vi "Control Panel.vi"(8 "error in (no error)":errorcluster, 11 "Fake Lakeshore Gaussmeter in":refnum<class "Lakeshore Gaussmeter.lvclass">) -> (0 "error out":errorcluster, 3 "Fake Lakeshore Gaussmeter out":refnum<class "Lakeshore Gaussmeter.lvclass">)   [LabVIEW 2017, in "Lakeshore Gaussmeter.lvclass"]
doc: "(Dynamic) A user-level application that simulates the physical front panel of the Instrument. Provide the user with buttons to manually control features of the instrument, and provide indicators of its current state."
uses:
  Lakeshore Gaussmeter.lvclass
  Lakeshore Gaussmeter.lvclass/Lakeshore Gaussmeter.ctl
  Utility Classes/Scannable/Scannable.lvclass
panel:
  in  "Auto Range Set (F: Off)":bool
  in  "Range Set (0: 1 - Lowest)":u16(ring) items=["1 - Lowest", "2", "3", "4", "5 - Highest"]
  out "Auto Range (F: Off)":bool
  out "Range (0: 1 - Lowest)":u16(ring) items=["1 - Lowest", "2", "3", "4", "5 - Highest"]
  in  "Set Units":bool
  in  "Field Control Mode Set":u16(ring) items=["Off", "Closed Loop PI", "Manual"]
  out "Field Control Mode":u16(ring) items=["Off", "Closed Loop PI", "Manual"]
  in  "Control Slope Limit Set (10.00000E+0)":dbl=10.0
  in  "Ramp Rate Set (3.50000E+3)":dbl=3500.0
  in  "Integral (reset) Set (1.00000E+0)":dbl=1.0
  in  "Proportional (gain) Set (10.00000E+0)":dbl=10.0
  in  "Setpoint Set":dbl min=0.0 max=13600.0
  out "Control Slope Limit":dbl
  out "Ramp Rate":dbl
  out "Integral (reset)":dbl
  out "Proportional (gain)":dbl
  out "Setpoint Ramping?":bool
  out "Setpoint":dbl
  in  "Field Units Set (0: Gauss)":u16(ring) items=["Gauss", "Tesla", "Oersted", "Amp/meter"]
  out "Field Units":u16(ring) items=["Gauss", "Tesla", "Oersted", "Amp/meter"]
  out "Field Reading":dbl
  in  "Reset":bool
  in  "Set Values":bool
  in  "Read to Control":bool
  in  "Read":bool
  in  "stop":bool
  in  "Copy actual to set":bool
  in  "Populate fields with member data":bool
  # "Not higher than 1.36T =13600G!"
  # "Inconsistent bug: set this to 10 in gauss mode (not 0.01) if field doesn't change when set."
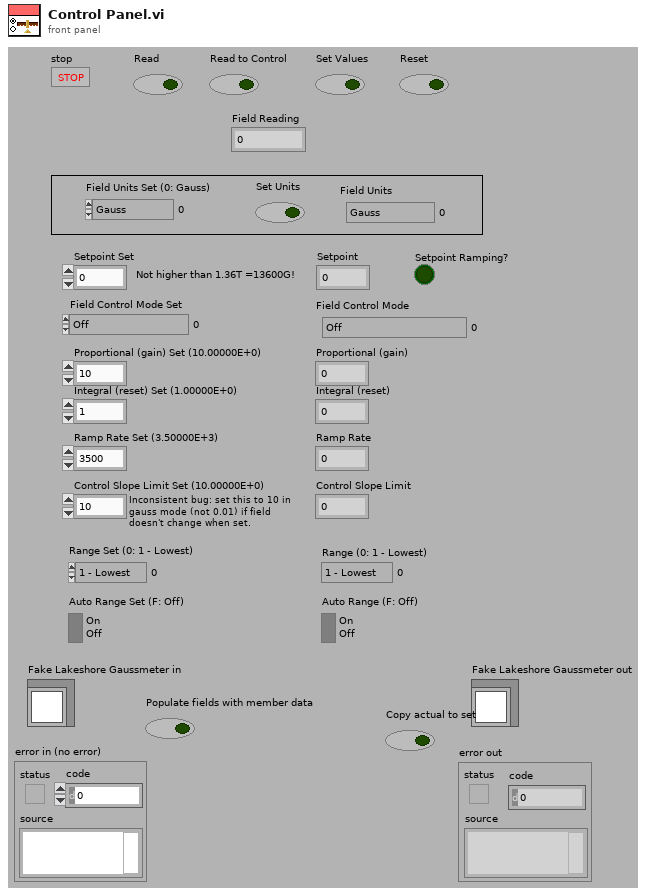
[diagram p1: front panel]
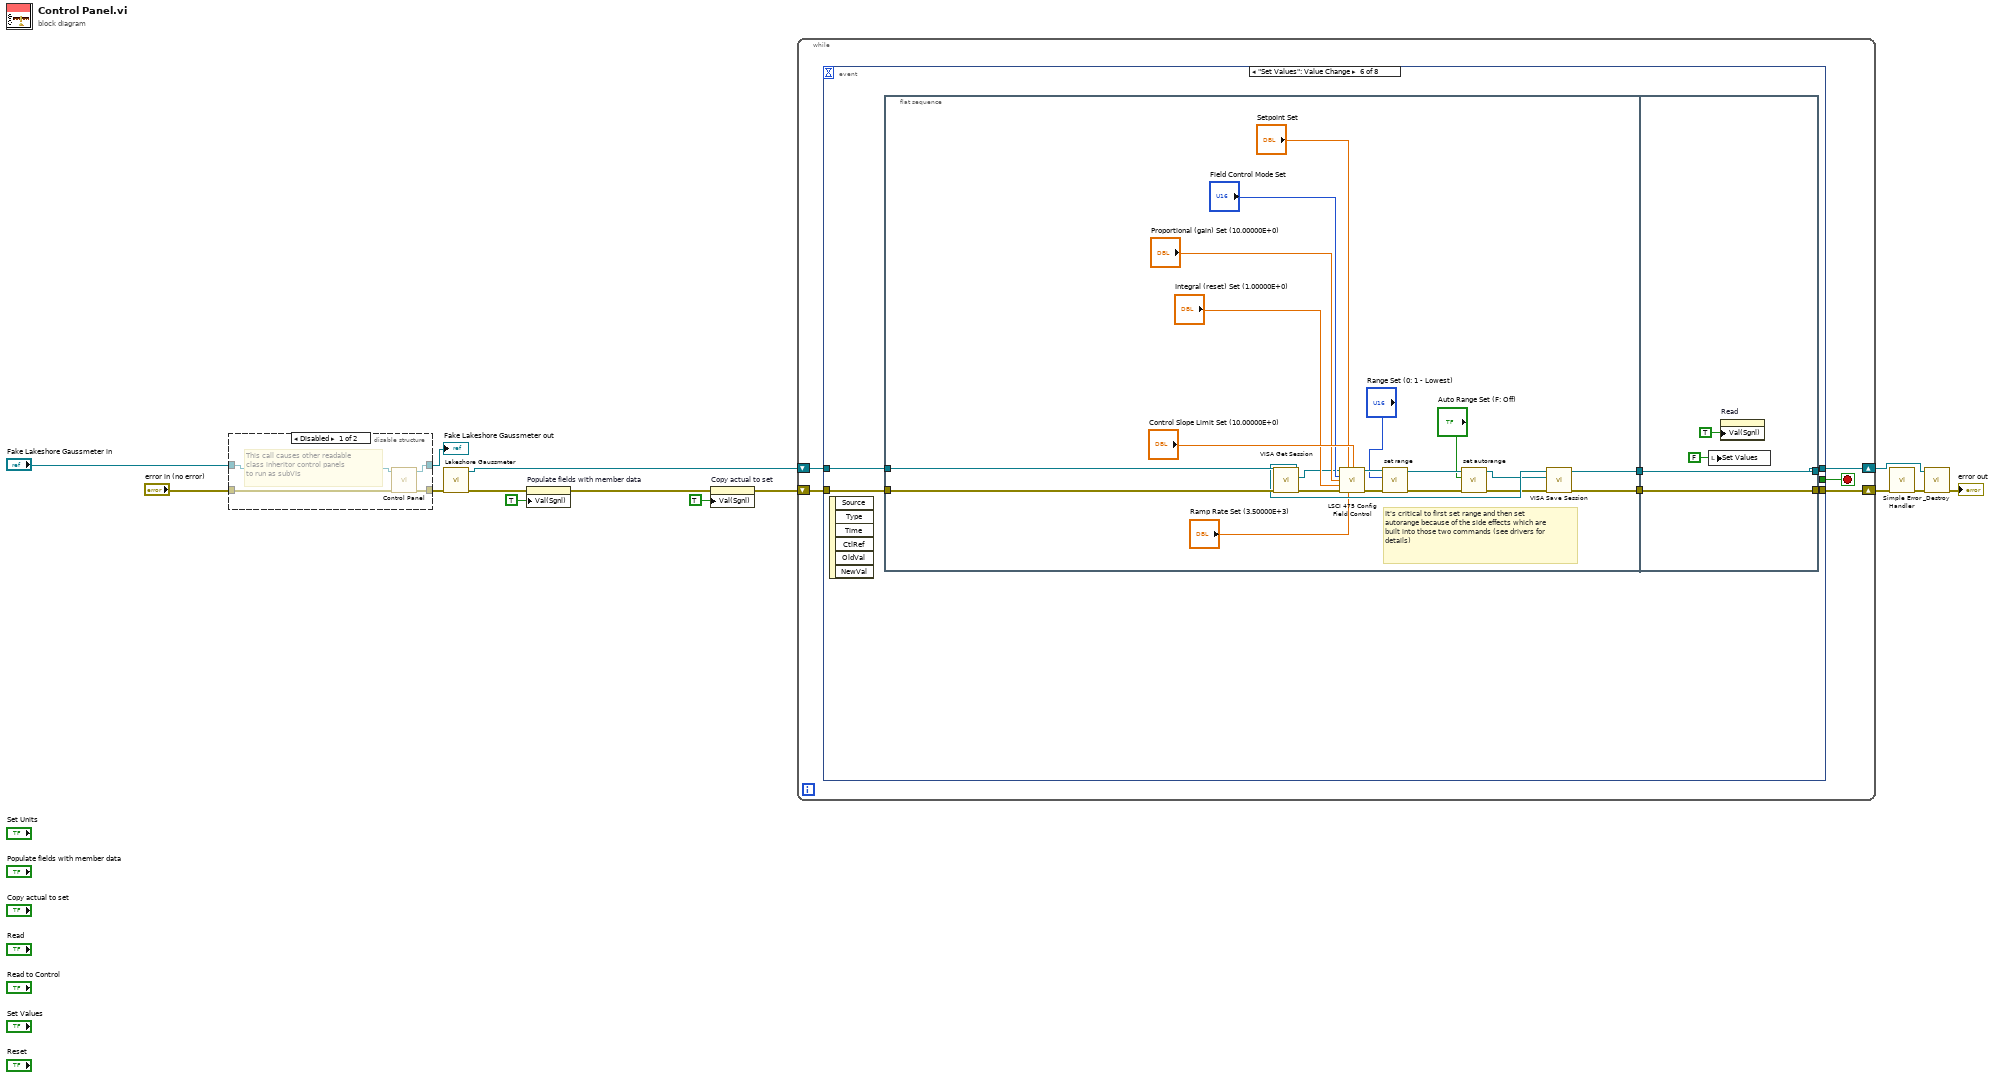
[diagram p0: block diagram]
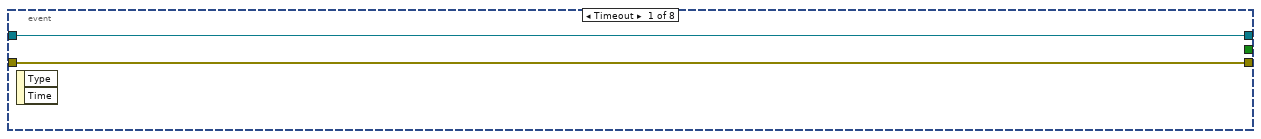
[diagram p3: hidden frame]
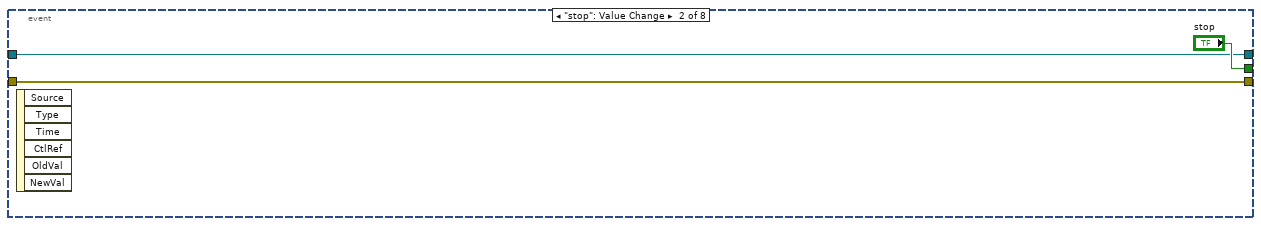
[diagram p4: hidden frame]
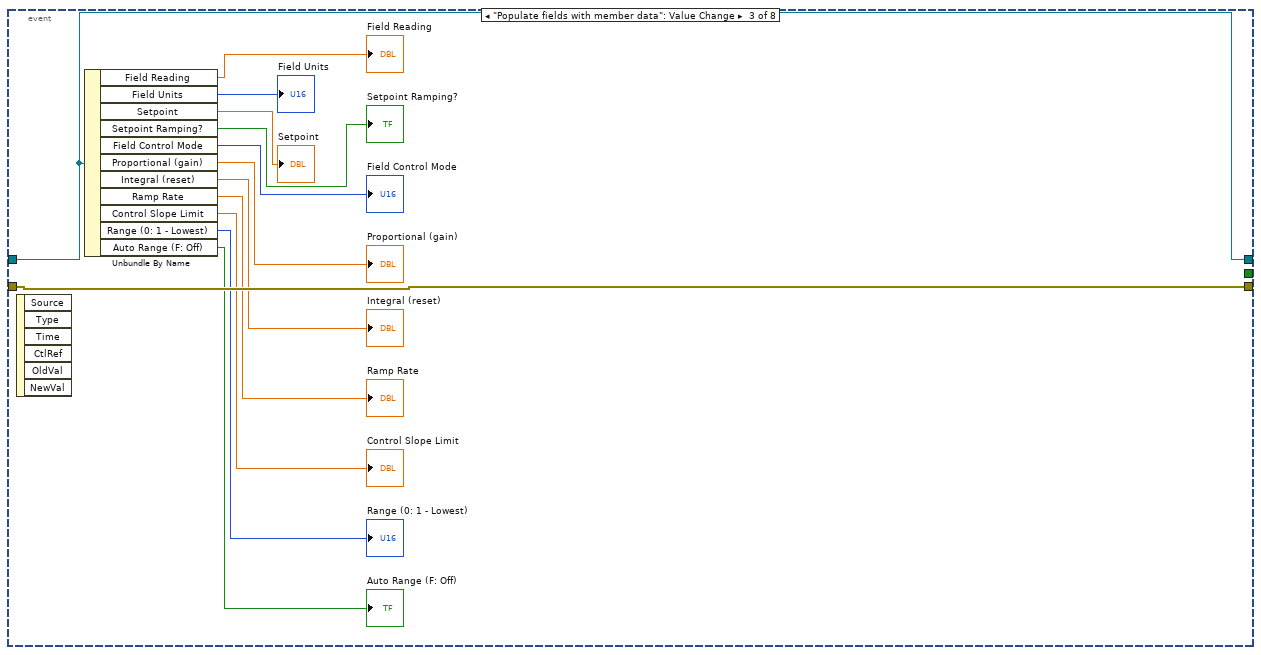
[diagram p5: hidden frame]
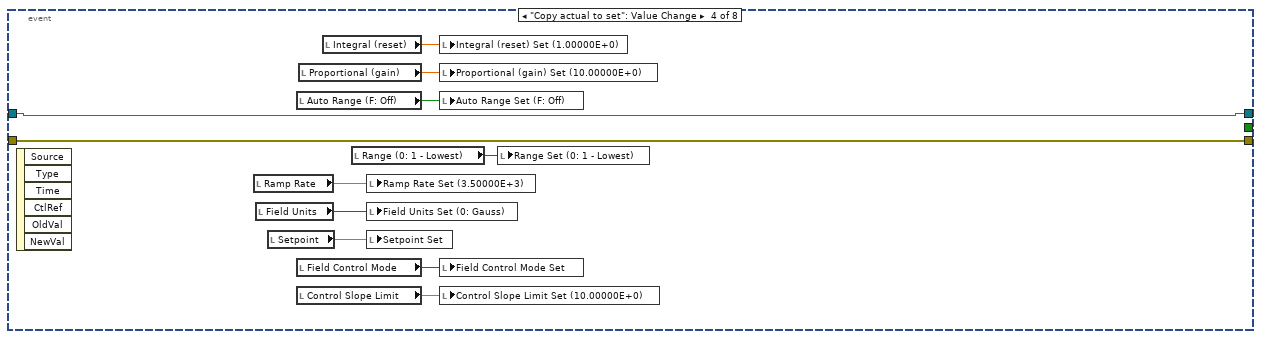
[diagram p6: hidden frame]
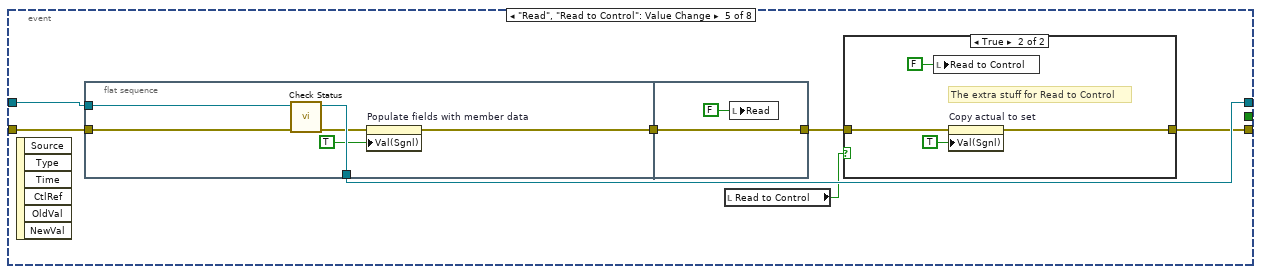
[diagram p7: hidden frame]
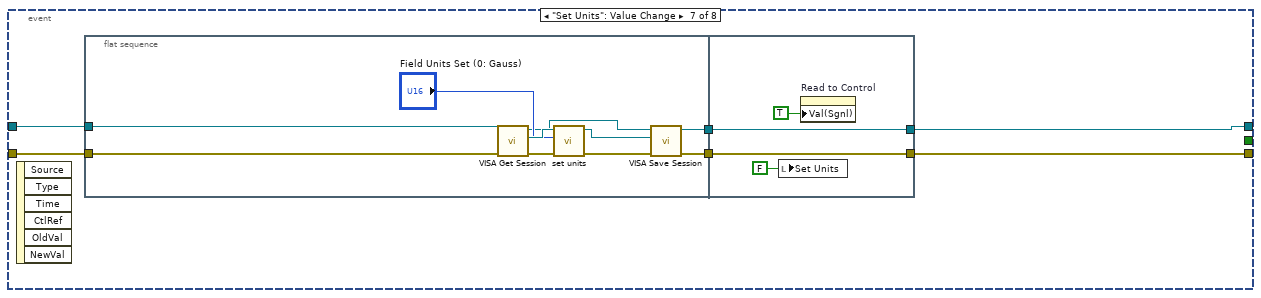
[diagram p9: hidden frame]
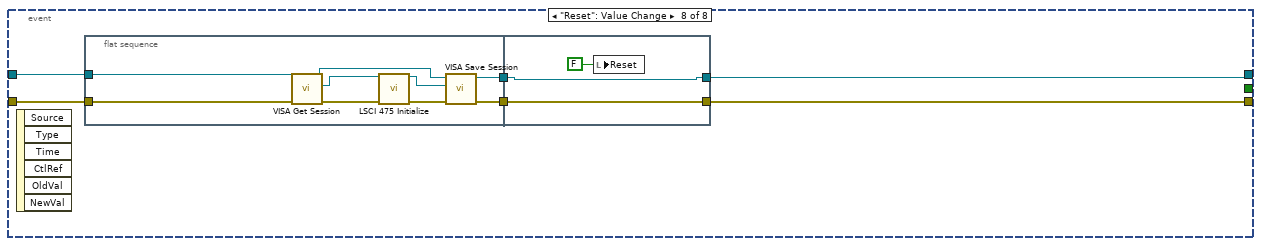
[diagram p10: hidden frame]
diagram:
  n1 = disable-structure shown="Disabled" {
    disable-tunnel: [w18 w19] -> w4
    disable-tunnel: [w17 w20] -> w14
    disable-tunnel: "error in (no error)" -> [w16 w19]
    disable-tunnel: "Fake Lakeshore Gaussmeter in" -> [w15 w20]
    frame Disabled {
      # "This call causes other readable\nclass inheritor control panels\nto run as subVIs"
      n2 = call-parent "Control Panel.vi"("error in (no error)"=w16, "Instrument in"=w15) -> ("error out"=w18:errorcluster, "Instrument out"=w17:refnum<class "Lakeshore Gaussmeter.lvclass">)  [unwired: 8 in]
    }
    frame Enabled {
    }
  }
  "Fake Lakeshore Gaussmeter out" <- w14
  n3 = call "Lakeshore Gaussmeter.vi"("error in (no error)"=w4) -> ("error out"=w2:errorcluster, "Lakeshore Gaussmeter out"=w3:refnum<class "Lakeshore Gaussmeter.lvclass">)  [unwired: 9 in]
  n4 = property on="Populate fields with member data" class="Bool (strict)"(error in=w2, "Val(Sgnl)"=TRUE ("Value (Signaling)")) -> (error out=w11:errorcluster)  [unwired: 1 in, 1 out]
  n5 = property on="Copy actual to set" class="Bool (strict)"(error in=w11, "Val(Sgnl)"=TRUE ("Value (Signaling)")) -> (error out=w10:errorcluster)  [unwired: 1 in, 1 out]
  n6 = while {
    shift-right: [w22] -> w9
    shift-left: w3 -> [w21]
    shift-right: [w24] -> w6
    shift-left: w10 -> [w23]
    stop <- w25 stop-if-true
    n7 = event shown="[5] \"Set Values\": Value Change" {
      selector: _ -> [_ _ _ _ _ _ _ _]
      dyn-events: _ -> [_ _ _ _ _ _ _ _]
      timeout: _ -> [_ _ _ _ _ _ _ _]
      tunnel: [_ "stop" _ _ _ _ _ _] -> w25
      tunnel: [w26 w29 w43 w53 w55 w77 w107 w129] -> w24
      tunnel: w23 -> [w26 w29 w43 w53 w61 w79 w110 w130]
      tunnel: [w27 w28 w42 w54 w59 w78 w108 w128] -> w22
      tunnel: w21 -> [w27 w28 w42 w54 w60 w80 w111 w131]
      event Timeout {
        n8 = event-data() -> ()  [unwired: 3 out]
      }
      event "stop": Value Change {
        n9 = event-data() -> ()  [unwired: 7 out]
      }
      event "Populate fields with member data": Value Change {
        n10 = event-data() -> ()  [unwired: 7 out]
        n11 = Unbundle By Name(w42) -> ("Field Reading"=→"Field Reading":dbl, "Field Units"=→"Field Units":u16, "Setpoint"=→"Setpoint":dbl, "Setpoint Ramping?"=→"Setpoint Ramping?":bool, "Field Control Mode"=→"Field Control Mode":u16, "Proportional (gain)"=→"Proportional (gain)":dbl, "Integral (reset)"=→"Integral (reset)":dbl, "Ramp Rate"=→"Ramp Rate":dbl, "Control Slope Limit"=→"Control Slope Limit":dbl, "Range (0: 1 - Lowest)"=→"Range (0: 1 - Lowest)":u16, "Auto Range (F: Off)"=→"Auto Range (F: Off)":bool)
      }
      event "Copy actual to set": Value Change {
        n12 = event-data() -> ()  [unwired: 7 out]
        n13 = local read "Ramp Rate"() -> (w47:dbl)
        n14 = local read "Field Units"() -> (w50:u16)
        n15 = local read "Setpoint"() -> (w46:dbl)
        n16 = local read "Auto Range (F: Off)"() -> (w44:bool)
        n17 = local read "Field Control Mode"() -> (w51:u16)
        n18 = local read "Control Slope Limit"() -> (w52:dbl)
        n19 = local read "Proportional (gain)"() -> (w48:dbl)
        n20 = local read "Integral (reset)"() -> (w49:dbl)
        n21 = local read "Range (0: 1 - Lowest)"() -> (w45:u16)
        n22 = local write "Ramp Rate Set (3.50000E+3)"(w47) -> ()
        n23 = local write "Field Units Set (0: Gauss)"(w50) -> ()
        n24 = local write "Setpoint Set"(w46) -> ()
        n25 = local write "Integral (reset) Set (1.00000E+0)"(w49) -> ()
        n26 = local write "Proportional (gain) Set (10.00000E+0)"(w48) -> ()
        n27 = local write "Auto Range Set (F: Off)"(w44) -> ()
        n28 = local write "Field Control Mode Set"(w51) -> ()
        n29 = local write "Control Slope Limit Set (10.00000E+0)"(w52) -> ()
        n30 = local write "Range Set (0: 1 - Lowest)"(w45) -> ()
      }
      event "Read", "Read to Control": Value Change {
        n31 = event-data() -> ()  [unwired: 7 out]
        n32 = flat-sequence {
          tunnel: w61 -> [w72]
          tunnel: w60 -> [w71]
          tunnel: [w70] -> w59
          tunnel: [w67] -> w56
          tunnel: [w73] -> w57
          tunnel: w56 -> [w73]
          frame #0 {
            n33 = call-dynamic "Check Status.vi"("error in (no error)"=w72, "Lakeshore Gaussmeter in"=w71) -> ("error out"=w69:errorcluster, "Lakeshore Gaussmeter out"=w70:refnum<class "Lakeshore Gaussmeter.lvclass">)  [unwired: 8 out]
            n34 = property on="Populate fields with member data" class="Bool (strict)"(error in=w69, "Val(Sgnl)"=TRUE ("Value (Signaling)")) -> (error out=w67:errorcluster)  [unwired: 1 in, 1 out]
          }
          frame #1 {
            n35 = local write "Read"(FALSE ("Read")) -> ()
          }
        }
        n36 = local read "Read to Control"() -> (w58:bool)
        n37 = case shown="True" w58 {
          tunnel: w57 -> [w62 w64]
          tunnel: [w62 w63] -> w55
          frame False {
          }
          frame True {
            # "The extra stuff for Read to Control"
            n38 = local write "Read to Control"(FALSE ("Read to Control")) -> ()
            n39 = property on="Copy actual to set" class="Bool (strict)"(error in=w64, "Val(Sgnl)"=TRUE ("Value (Signaling)")) -> (error out=w63:errorcluster)  [unwired: 1 in, 1 out]
          }
        }
      }
      event "Set Values": Value Change {
        n40 = event-data() -> ()  [unwired: 7 out]
        n41 = flat-sequence {
          tunnel: w80 -> [w101]
          tunnel: w79 -> [w100]
          tunnel: [w98] -> w76
          tunnel: [w97] -> w75
          tunnel: [w104] -> w77
          tunnel: [w105] -> w78
          tunnel: w76 -> [w105]
          tunnel: w75 -> [w104]
          frame #0 {
            # "It's critical to first set range and then set autorange because of the side effects which are built into those two commands (see drivers for details)"
            n42 = call-dynamic "VISA Get Session.vi"("error in (no error)"=w100, "Instrument.lvclass in"=w101) -> ("error out"=w89:errorcluster, "VISA Resource Name"=w90:refnum<visa-resource-name>, "Instrument.lvclass out"=w99:refnum<class "Lakeshore Gaussmeter.lvclass">)  [unwired: 7 out]
            n43 = call "LSCI 475 Config Field Control.vi"("VISA session"=w90, "Setpoint (0.00000E+0)"="Setpoint Set", "Control Slope Limit (10.00000E+0)"="Control Slope Limit Set (10.00000E+0)", "Field Control Mode (0: Off)"="Field Control Mode Set", "Proportional (gain) (10.00000E+0)"="Proportional (gain) Set (10.00000E+0)", "Integral (reset) (1.00000E+0)"="Integral (reset) Set (1.00000E+0)", "error in (no error)"=w89, "Ramp Rate (3.50000E+3)"="Ramp Rate Set (3.50000E+3)") -> ("dup VISA session"=w87:refnum<visa-resource-name>, "error out"=w88:errorcluster)  [unwired: 6 in]
            n44 = call "set range.vi"("error in (no error)"=w88, "Range (0: 1 - Lowest)"="Range Set (0: 1 - Lowest)", "VISA session"=w87) -> ("error out"=w86:errorcluster, "dup VISA session"=w85:refnum<visa-resource-name>)  [unwired: 7 in]
            n45 = call "set autorange.vi"("error in (no error)"=w86, "Auto Range (F: Off)"="Auto Range Set (F: Off)", "VISA session"=w85) -> ("error out"=w83:errorcluster, "dup VISA session"=w84:refnum<visa-resource-name>)  [unwired: 7 in]
            n46 = call-dynamic "VISA Save Session.vi"("error in (no error)"=w83, "VISA Resource Name"=w84, "Instrument.lvclass in"=w99) -> ("error out"=w97:errorcluster, "Instrument.lvclass out"=w98:refnum<class "Lakeshore Gaussmeter.lvclass">)  [unwired: 7 out]
          }
          frame #1 {
            n47 = local write "Set Values"(FALSE ("Set")) -> ()
            n48 = property on="Read" class="Bool (strict)"("Val(Sgnl)"=TRUE ("Value (Signaling)")) -> ()  [unwired: 2 in, 2 out]
          }
        }
      }
      event "Set Units": Value Change {
        n49 = event-data() -> ()  [unwired: 7 out]
        n50 = flat-sequence {
          tunnel: w111 -> [w121]
          tunnel: w110 -> [w120]
          tunnel: [w119] -> w109
          tunnel: [w118] -> w106
          tunnel: w109 -> [w123]
          tunnel: [w123] -> w108
          tunnel: [w122] -> w107
          tunnel: w106 -> [w122]
          frame #0 {
            n51 = call-dynamic "VISA Get Session.vi"("error in (no error)"=w120, "Instrument.lvclass in"=w121) -> ("error out"=w115:errorcluster, "VISA Resource Name"=w117:refnum<visa-resource-name>, "Instrument.lvclass out"=w112:refnum<class "Lakeshore Gaussmeter.lvclass">)  [unwired: 7 out]
            n52 = call "set units.vi"("error in (no error)"=w115, "Field Units (0: Gauss)"="Field Units Set (0: Gauss)", "VISA session"=w117) -> ("error out"=w113:errorcluster, "dup VISA session"=w114:refnum<visa-resource-name>)  [unwired: 7 in]
            n53 = call-dynamic "VISA Save Session.vi"("error in (no error)"=w113, "VISA Resource Name"=w114, "Instrument.lvclass in"=w112) -> ("error out"=w118:errorcluster, "Instrument.lvclass out"=w119:refnum<class "Lakeshore Gaussmeter.lvclass">)  [unwired: 7 out]
          }
          frame #1 {
            n54 = local write "Set Units"(FALSE ("Set")) -> ()
            n55 = property on="Read to Control" class="Bool (strict)"("Val(Sgnl)"=TRUE ("Value (Signaling)")) -> ()  [unwired: 2 in, 2 out]
          }
        }
      }
      event "Reset": Value Change {
        n56 = event-data() -> ()  [unwired: 7 out]
        n57 = flat-sequence {
          tunnel: w131 -> [w140]
          tunnel: w130 -> [w139]
          tunnel: [w137] -> w127
          tunnel: [w136] -> w126
          tunnel: [w142] -> w128
          tunnel: [w143] -> w129
          tunnel: w127 -> [w143]
          tunnel: w126 -> [w142]
          frame #0 {
            n58 = call-dynamic "VISA Get Session.vi"("error in (no error)"=w139, "Instrument.lvclass in"=w140) -> ("error out"=w133:errorcluster, "VISA Resource Name"=w135:refnum<visa-resource-name>, "Instrument.lvclass out"=w138:refnum<class "Lakeshore Gaussmeter.lvclass">)  [unwired: 7 out]
            n59 = call "LSCI 475 Initialize.vi"("VISA Resource Name"=w135, "error in (no error)"=w133) -> ("VISA session"=w134:refnum<visa-resource-name>, "error out"=w132:errorcluster)  [unwired: 12 in]
            n60 = call-dynamic "VISA Save Session.vi"("error in (no error)"=w132, "VISA Resource Name"=w134, "Instrument.lvclass in"=w138) -> ("error out"=w137:errorcluster, "Instrument.lvclass out"=w136:refnum<class "Lakeshore Gaussmeter.lvclass">)  [unwired: 7 out]
          }
          frame #1 {
            n61 = local write "Reset"(FALSE ("Read to Control")) -> ()
          }
        }
      }
    }
  }
  n62 = call <vilib>:"Simple Error Handler.vi"("error in (no error)"=w6) -> ("error out"=w5:errorcluster)  [unwired: 1 in, 7 out]
  n63 = call-dynamic "_Destroy.vi"("error in (no error)"=w5, "Instrument in"=w9) -> ("error out"=→"error out":errorcluster)  [unwired: 9 out]
